vi "Calibration from image (SubVI).vi"(8 "error in (no error)":errorcluster, 11 "Refnum in":T1) -> (0 "error out":errorcluster, 3 "Refnum out":T1)   [LabVIEW 2013]
uses:
  <vilib>/vision/Image Controls.llb/IMAQ Image.ctl
  <vilib>/vision/NI_Vision_Development_Module.lvlib
  <vilib>/Utility/file.llb/Write To Spreadsheet File (DBL).vi
panel:
  out "Error Map":sgl[][](array[numeric]) format="%.2f"
  out "Image":T1(plugin-control)
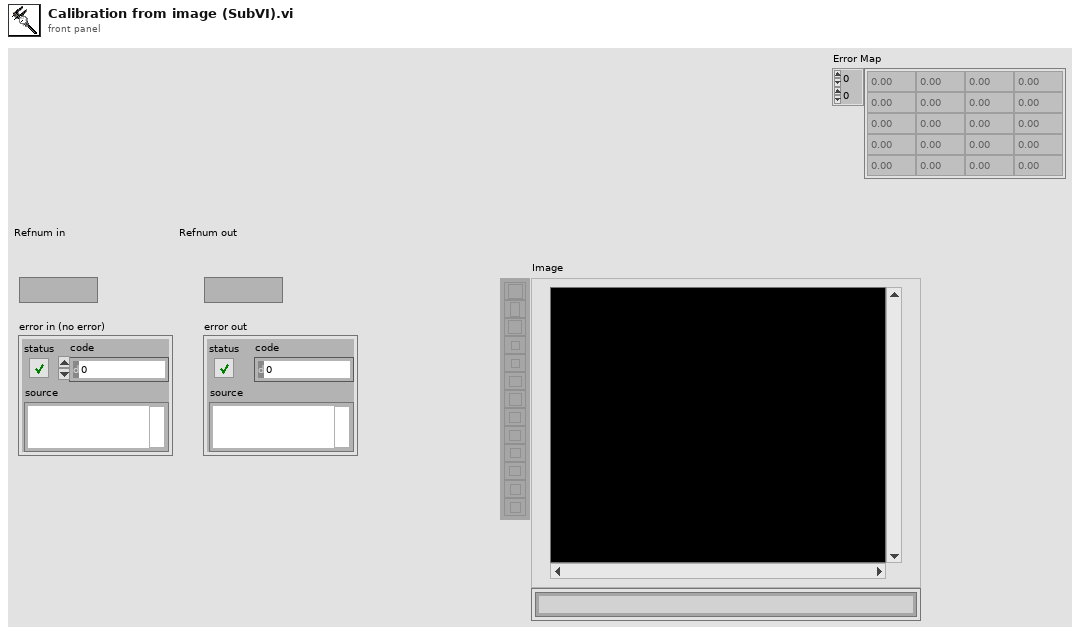
[diagram p1: front panel]
types:
  T1 = typedef "IMAQ Image.ctl" = refnum<image>
  T2 = typedef "Image Type" = u32
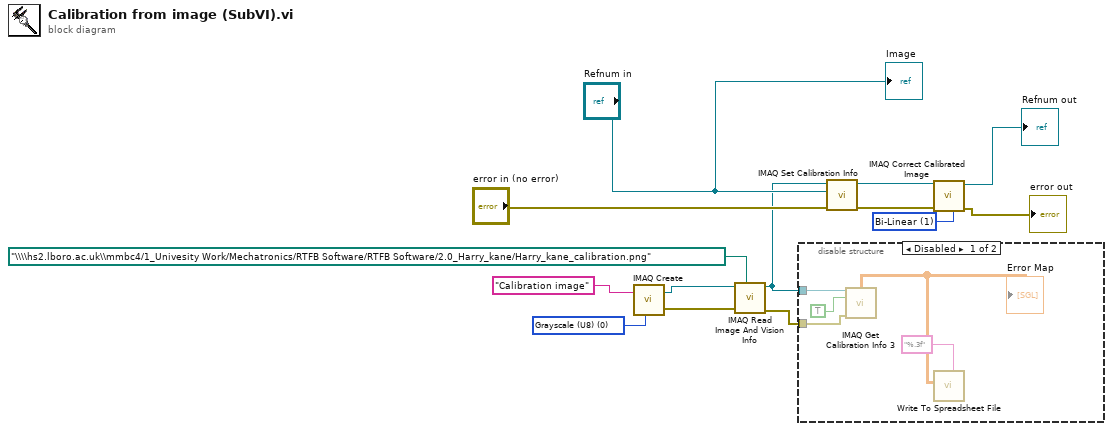
[diagram p0: block diagram]
diagram:
  w10 = T2 0 items=["Grayscale (U8)", "Grayscale (I16)", "Grayscale (SGL)", "Complex (CSG)", "RGB (U32)", "HSL (U32)", "RGB (U64)", "Grayscale (U16)"] ("Image Type")
  w11 = u32 1 items=["Zero Order", "Bi-Linear", "Quadratic", "Cubic Spline"] ("Interpolation Type")
  n1 = call "IMAQ Create"("Image Name"="Calibration image", "Image Type"=w10) -> ("New Image"=w6:T1, "error out"=w7:errorcluster)  [unwired: 3 in]
  n2 = call "IMAQ Read Image And Vision Info"("File Path"=path "\\\\hs2.lboro.ac.uk\\mmbc4/1_Univesity Work/Mechatronics/RTFB Software/RTFB Software/2.0_Harry_kane/Harry_kane_calibration.png", "error in (no error)"=w7, "Image"=w6) -> ("error out"=w3:errorcluster, "Image Out"=w2:T1)  [unwired: 6 in, 1 out]
  n3 = disable-structure shown="Disabled" {
    disable-tunnel: w2 -> [w19 _]
    disable-tunnel: w3 -> [w17 _]
    frame Disabled {
      n4 = call "IMAQ Get Calibration Info 3"("Calibration Template Image"=w19, "Return Error Information (False)"=TRUE, "error in (no error)"=w17) -> ("Error Map"=w16:sgl[][])  [unwired: 4 in, 8 out]
      "Error Map" <- w16
      n5 = call-poly <vilib>:"Write To Spreadsheet File.vi"("format (%.3f)"="%.3f", "2D data"=w16) -> ()  [unwired: 6 in, 1 out]
    }
    frame Enabled {
    }
  }
  n6 = call "IMAQ Set Calibration Info"("error in (no error)"="error in (no error)", "Image Dst"="Refnum in", "Image Src"=w2) -> ("error out"=w12:errorcluster, "Calibrated Image"=w8:T1)  [unwired: 7 in]
  n7 = call "IMAQ Correct Calibrated Image"("Interpolation Type"=w11, "error in (no error)"=w12, "Image Src"=w8) -> ("error out"=→"error out":errorcluster, "Corrected Image"=→"Refnum out":T1)  [unwired: 7 in]
  "Image" <- "Refnum in"
